vi "value to ring (Strobe).vi"(11 "value":string) -> (3 "Strobe":u32)   [LabVIEW 2020, in "AIM ARINC 664 Import.lvlib"]
uses:
  AIM ARINC 664 Import.lvlib
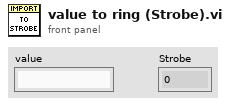
[diagram p1: front panel]
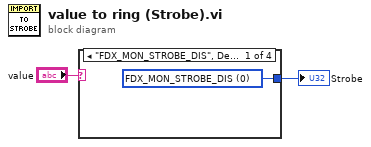
[diagram p0: block diagram]
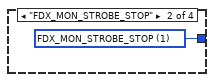
[diagram p2: hidden frame]
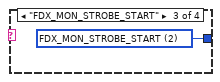
[diagram p3: hidden frame]
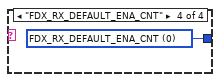
[diagram p4: hidden frame]
diagram:
  n1 = case shown="\"FDX_MON_STROBE_DIS\", Default" "value" {
    tunnel: [w3 w4 w5 w6] -> w2
    frame "FDX_MON_STROBE_DIS", Default {
      w3 = u32 0 items=["FDX_MON_STROBE_DIS", "FDX_MON_STROBE_STOP", "FDX_MON_STROBE_START"] ("Strobe")
    }
    frame "FDX_MON_STROBE_STOP" {
      w4 = u32 1 items=["FDX_MON_STROBE_DIS", "FDX_MON_STROBE_STOP", "FDX_MON_STROBE_START"] ("Strobe")
    }
    frame "FDX_MON_STROBE_START" {
      w5 = u32 2 items=["FDX_MON_STROBE_DIS", "FDX_MON_STROBE_STOP", "FDX_MON_STROBE_START"] ("Strobe")
    }
    frame "FDX_RX_DEFAULT_ENA_CNT" {
      w6 = u32 0 items=["FDX_RX_DEFAULT_ENA_CNT", "FDX_RX_DEFAULT_MON_ENA_ALL", "FDX_RX_DEFAULT_MON_ENA_GOOD"] ("DefaultCronoMode")
    }
  }
  "Strobe" <- w2
